vi "删除文件夹.vi"(0 "产品型号路径":path, 5 "产品型号":string="potteryTemplete", 11 "error in (no error)":errorcluster caption="错误输入（无错误）") -> (15 "error out":errorcluster caption="错误输出")   [LabVIEW 2017]
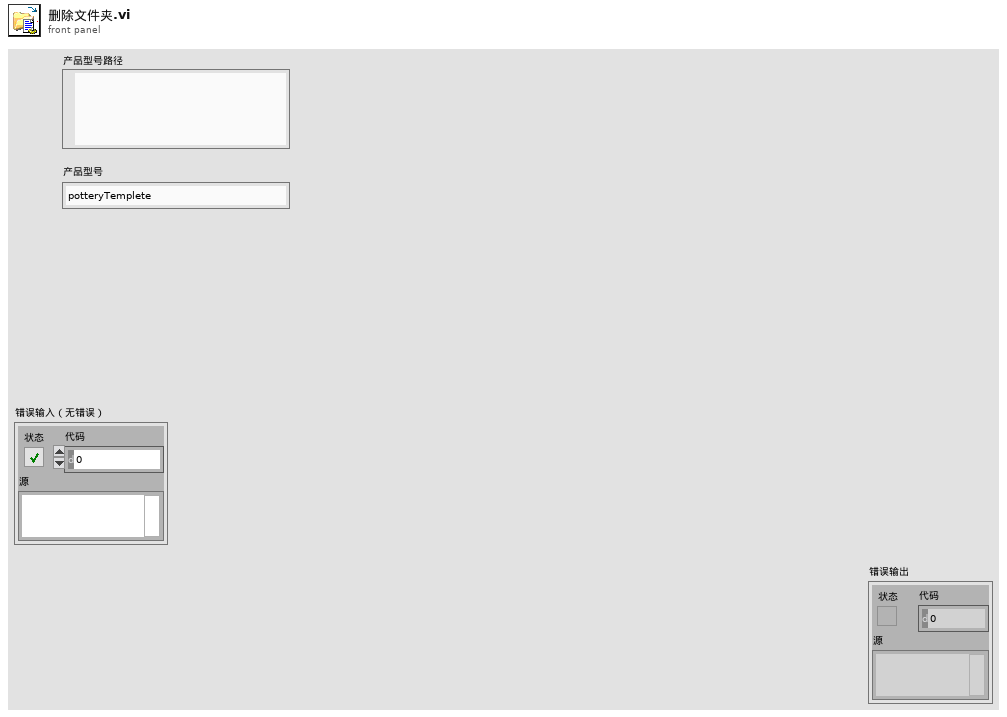
[diagram p1: front panel]
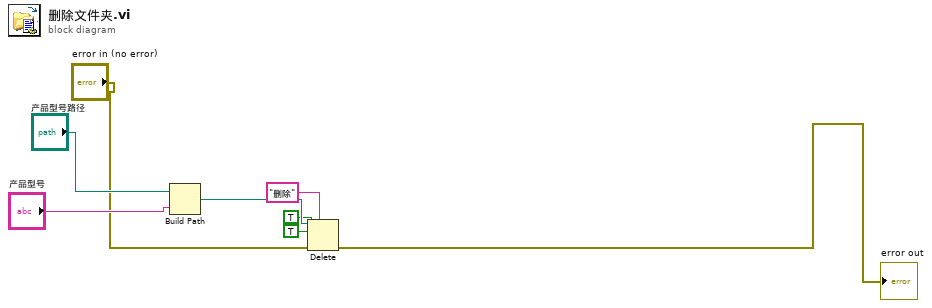
[diagram p0: block diagram]
diagram:
  n1 = Build Path(base path="产品型号路径", name or relative path="产品型号") -> (appended path=w6:path)
  n2 = Delete(prompt (Delete)="删除" ("对话框窗口（选择或输入文件路径）"), path (use dialog)=w6, entire hierarchy (F)=TRUE ("整个层次结构(F)"), confirm (F)=TRUE ("确认(F)"), error in="error in (no error)") -> (error out=→"error out":errorcluster)  [unwired: 2 out]
